vi "Builder.vi"(8 "error in (no error)":errorcluster, 10 "Map":i32[](array[numeric]), 11 "Builder In":refnum<class "Cross.lvclass">) -> (0 "error out":errorcluster, 1 "Direction":T1, 2 "Action":T2, 3 "Builder Out":refnum<class "Cross.lvclass">, 4 "Replicated Class":refnum<class "Cross.lvclass">)   [LabVIEW 2015, in "Cross.lvclass"]
uses:
  Cross.lvclass
  Type Defs/Action Enum.ctl
  Type Defs/Direction Enum.ctl
  Cross.lvclass/Cross.ctl
  Type Defs/SB Type Defs.lvlib
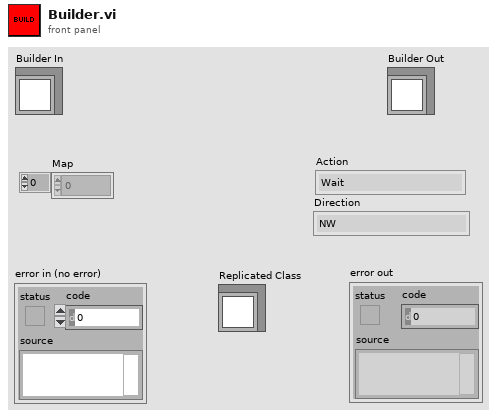
[diagram p1: front panel]
types:
  T1 = typedef "SB Type Defs.lvlib/Direction Enum.ctl" = enum16{"NW", "N", "NE", "E", "SE", "S", "SW", "W"}
  T2 = typedef "SB Type Defs.lvlib/Action Enum.ctl" = enum16{"Wait", "Move", "Attack", "Replicate"}
  T3 = enum16{"Raw", "Spawner", "Builder", "Gunner", "Fighter"}
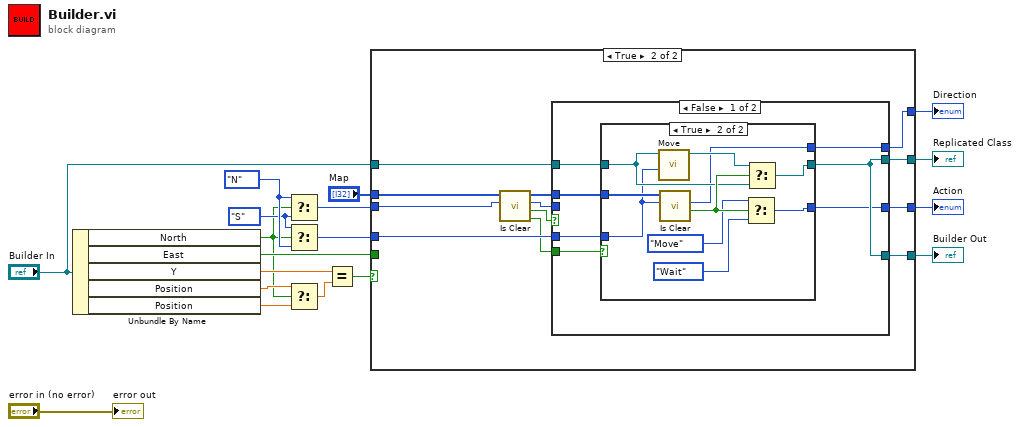
[diagram p0: block diagram]
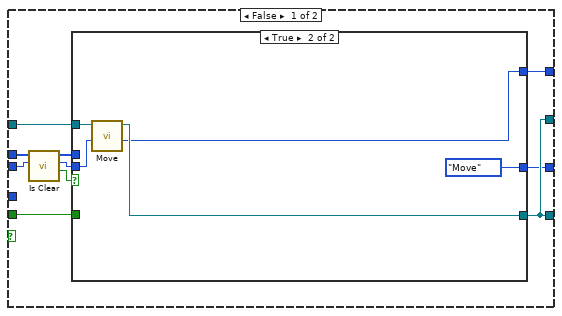
[diagram p2: hidden frame]
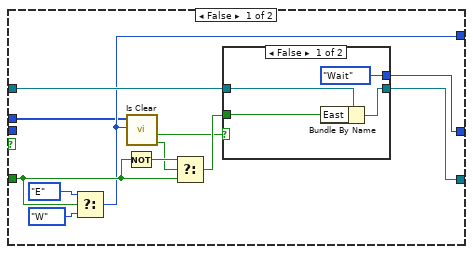
[diagram p3: hidden frame]
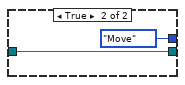
[diagram p4: hidden frame]
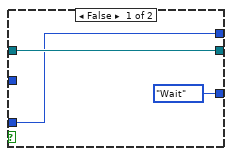
[diagram p5: hidden frame]
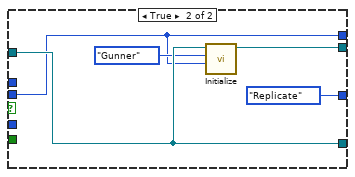
[diagram p6: hidden frame]
diagram:
  w9 = Direction_Enum."S" ("Direction")
  w10 = Direction_Enum."N" ("Direction")
  n1 = Unbundle By Name("Builder In") -> ("North"=w1:bool, "East"=w12:bool, "Y"=w2:dbl, "Position"=w8:dbl, "Position"=w7:dbl)
  n2 = Select(t=w10, s=w1, f=w9) -> (s? t:f=w4:T1)
  n3 = Select(t=w9, s=w1, f=w10) -> (s? t:f=w3:T1)
  n4 = Select(t=w8, s=w1, f=w7) -> (s? t:f=w6:dbl)
  n5 = Equal?(x=w2, y=w6) -> (x = y?=w5:bool)
  n6 = case shown="True" w5 {
    tunnel: [w25 w58] -> w17
    tunnel: "Builder In" -> [w28 w57]
    tunnel: [w27 w55] -> w15
    tunnel: [w27 w56] -> w14
    tunnel: [w26 w53] -> w13
    tunnel: w12 -> [w24 _]
    tunnel: "Map" -> [w23 w63]
    tunnel: w4 -> [w19 w62]
    tunnel: w3 -> [_ w59]
    frame False {
      n7 = call "Is Clear.vi"("Direction"=w19, "Maze"=w23) -> ("Can Move?"=w21:bool, "Direction Out"=w20:T1, "Maze"=w22:i32[])  [unwired: 6 in, 1 out]
      n8 = case shown="True" w21 {
        tunnel: w28 -> [w36 w50]
        tunnel: [w35 w49] -> w27
        tunnel: [w31 w47] -> w26
        tunnel: [w34 Action_Enum."Move" ("Action")] -> w25
        tunnel: w22 -> [w29 _]
        tunnel: w24 -> [w33 _]
        tunnel: w20 -> [_ w48]
        frame False {
          n9 = Select(t=Direction_Enum."E" ("Direction"), s=w33, f=Direction_Enum."W" ("Direction")) -> (s? t:f=w31:T1)
          n10 = Not(x=w33) -> (.not. x?=w40:bool)
          n11 = call "Is Clear.vi"("Direction"=w31, "Maze"=w29) -> ("Blocked?"=w30:bool, "Can Move?"=w32:bool)  [unwired: 6 in, 2 out]
          n12 = Select(t=w40, s=w30, f=w33) -> (s? t:f=w39:bool)
          n13 = case shown="False" w32 {
            tunnel: [Action_Enum."Wait" ("Action") Action_Enum."Move" ("Action")] -> w34
            tunnel: w36 -> [w41 w45]
            tunnel: w39 -> [w42 _]
            tunnel: [w43 w45] -> w35
            frame False {
              n14 = Bundle By Name(cluster=w41, "East"=w42) -> (w43:refnum<class "Cross.lvclass">)
            }
            frame True {
            }
          }
        }
        frame True {
          n15 = call "Move.vi"("Direction"=w48, "Cross.lvclass"=w50) -> ("Direction 2"=w47:T1, "Cross.lvclass 2"=w49:refnum<class "Cross.lvclass">)  [unwired: 8 in]
        }
      }
    }
    frame True {
      n16 = call "Is Clear.vi"("Direction"=w62, "Maze"=w63) -> ("Blocked?"=w52:bool, "Can Move?"=w61:bool, "Direction Out"=w54:T1, "Maze"=w60:i32[])  [unwired: 6 in]
      n17 = case shown="False" w61 {
        tunnel: w60 -> [w67 _]
        tunnel: w59 -> [w66 _]
        tunnel: [w64 Action_Enum."Replicate" ("Action")] -> w58
        tunnel: w57 -> [w69 w88]
        tunnel: [w68 w88] -> w55
        tunnel: [w68 w87] -> w56
        tunnel: w54 -> [_ w84]
        tunnel: [w65 w84] -> w53
        tunnel: w52 -> [w70 _]
        frame False {
          n18 = case shown="True" w70 {
            tunnel: w69 -> [w72 w79]
            tunnel: [w72 w78] -> w68
            tunnel: w67 -> [_ w77]
            tunnel: w66 -> [w71 w76]
            tunnel: [w71 w75] -> w65
            tunnel: [Action_Enum."Wait" ("Action") w74] -> w64
            frame False {
            }
            frame True {
              n19 = call "Move.vi"("Direction"=w76, "Cross.lvclass"=w79) -> ("Cross.lvclass 2"=w82:refnum<class "Cross.lvclass">)  [unwired: 8 in, 1 out]
              n20 = call "Is Clear.vi"("Direction"=w76, "Maze"=w77) -> ("Can Move?"=w83:bool, "Direction Out"=w75:T1)  [unwired: 6 in, 2 out]
              n21 = Select(t=Action_Enum."Move" ("Action"), s=w83, f=Action_Enum."Wait" ("Action")) -> (s? t:f=w74:T2)
              n22 = Select(t=w82, s=w83, f=w79) -> (s? t:f=w78:refnum<class "Cross.lvclass">)
            }
          }
        }
        frame True {
          n23 = call "Initialize.vi"("Direction"=w84, "Job"=T3."Gunner", "Runner in"=w88) -> ("Runner out"=w87:refnum<class "Cross.lvclass">)  [unwired: 8 in]
        }
      }
    }
  }
  "Action" <- w17
  "Direction" <- w13
  "Replicated Class" <- w14
  "Builder Out" <- w15
  "error out" <- "error in (no error)"
